vi "CMD Step 2 Digits of Significance.vi"(0 "CMD Step":dbl format="%#_13g") -> (4 "Digits of Significance":i32)   [LabVIEW 2013]
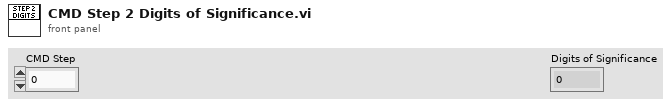
[diagram p1: front panel]
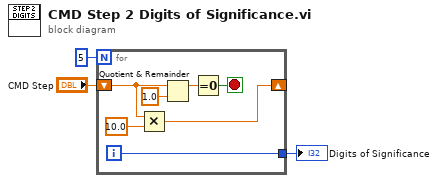
[diagram p0: block diagram]
diagram:
  n1 = for {
    N: 5 -> [_]
    shift-right: [w4] -> _
    shift-left: "CMD Step" -> [w6]
    tunnel: [w7] -> w2
    i -> [w7]
    stop <- w8 stop-if-true
    n2 = Multiply(x=w6, y=10.0) -> (x*y=w4:dbl)
    n3 = Quotient & Remainder(x=w6, y=1.0) -> (x-y*floor(x/y)=w9:dbl)  [unwired: 1 out]
    n4 = Equal To 0?(x=w9) -> (x = 0?=w8:bool)
  }
  "Digits of Significance" <- w2
